vi "SwissSPAD Live_Get Queue.vi"(4 "create if not found? (F)":bool) -> (5 "error out":errorcluster, 7 "SwissSPAD Queue":refnum<queue>)   [LabVIEW 2021]
uses:
  SwissSPAD Live_Q [Element].ctl
  SwissSPAD Live_Q Event List.ctl
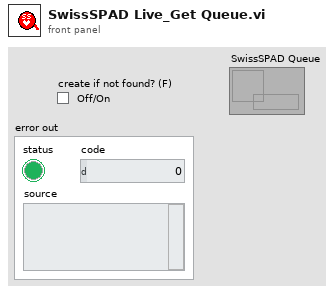
[diagram p1: front panel]
types:
  T1 = typedef "SwissSPAD Live_Q [Element].ctl" = cluster{"SwissSPAD Q Event":T2, "Data":variant}
  T2 = typedef "SwissSPAD Live_Q Event List.ctl" = enum16{"---- UI ----", "Idle", "Initialization", "Init FPGA(s)", "Init Top FPGA (deprecated)", "FPGA(s) Status", "Top FPGA Status (deprecated)", "Reset FPGA(s)", "Reset Top FPGA (deprecated)", "Refresh Display Image", "Quit", "---- DAQ ----", "Start Recording", "Start Live Acquisition", "Initialize Recording Mode", "Initialize FPGA (Live Mode)", "Get Image Set", "Get Single Image", "Update Image Display", "Stop Live Acquisition", "Stop Data Recording", "Stop Data Saving", "---- Image ----", "Copy Data to Clipboard", "Set Image Palette", "Save Displayed Image with Overlay", "Save Image Data as TIFF"}
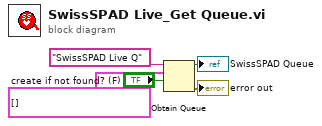
[diagram p0: block diagram]
diagram:
  n1 = Obtain Queue(name (unnamed)="SwissSPAD Live Q", element data type=T1[] [] ("element"), create if not found? (T)="create if not found? (F)") -> (queue out=→"SwissSPAD Queue":refnum<queue>, error out=→"error out":errorcluster)  [unwired: 2 in, 1 out]
